vi "Boiler Controller.vi"(8 "error in":errorcluster, 10 "Notifiers":T1, 11 "Message Queues":T2) -> (0 "error out":errorcluster)   [LabVIEW 2026]
uses:
  support/Message Queue/All Message Queues.ctl
  support/Message Queue/Message Cluster.ctl
  support/Notifiers/Notifiers.ctl
  support/Message Queue/Message Queue.lvlib
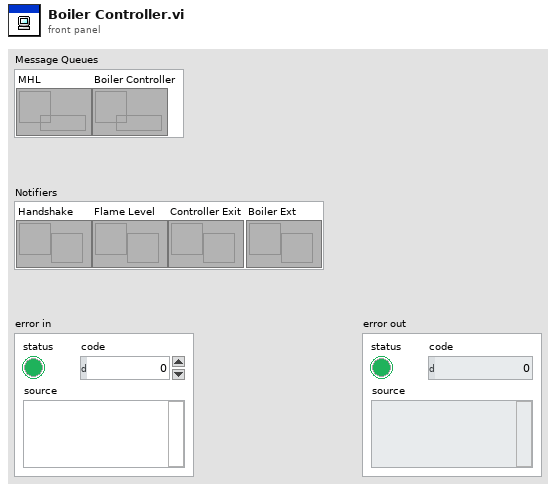
[diagram p1: front panel]
types:
  T1 = typedef "Notifiers.ctl" = cluster{"Handshake":refnum<notifier>, "Flame Level":refnum<notifier>, "Controller Exit":refnum<notifier>, "Boiler Ext":refnum<notifier>}
  T2 = typedef "Message Queue.lvlib/All Message Queues.ctl" = cluster{"MHL":refnum<queue>, "Boiler Controller":refnum<queue>}
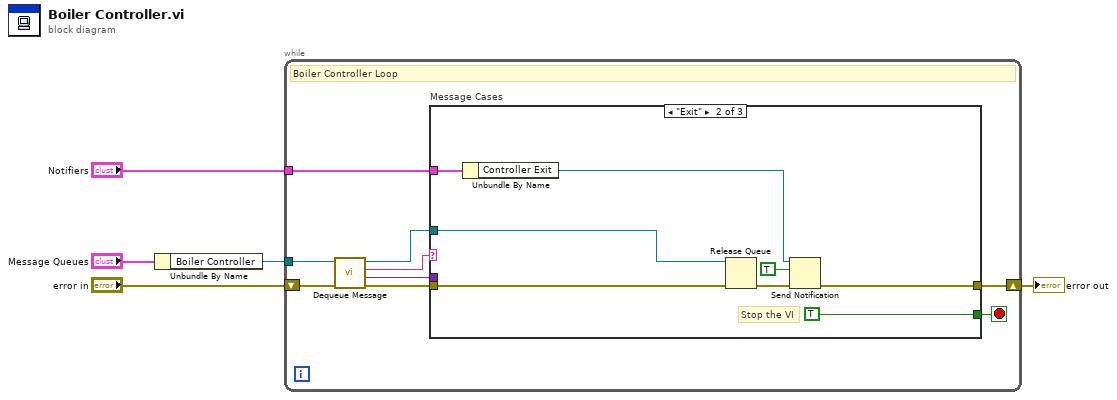
[diagram p0: block diagram]
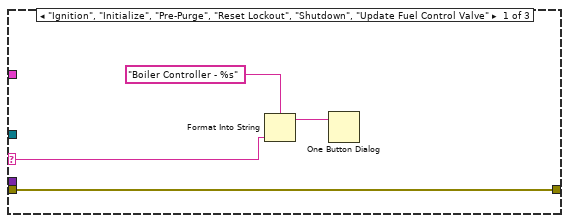
[diagram p2: hidden frame]
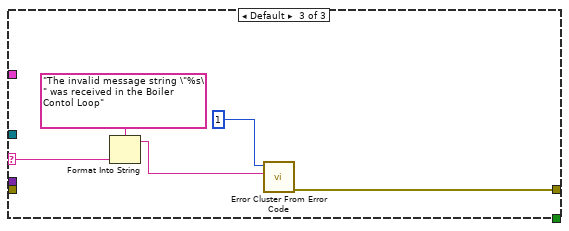
[diagram p3: hidden frame]
diagram:
  n1 = Unbundle By Name("Message Queues") -> ("Boiler Controller"=w3:refnum<queue>)
  n2 = while {
    tunnel: w3 -> [w11]
    shift-right: [w12] -> w4
    shift-left: "error in" -> [w13]
    tunnel: "Notifiers" -> [w6]
    stop <- w7 stop-if-true
    # "Boiler Controller Loop"
    n3 = call "Dequeue Message.vi"("error in"=w13, "Message Queue"=w11) -> ("error out"=w14:errorcluster, "Message Data"=w8:variant, "Message"=w10:string, "dup Message Queue"=w9:refnum<queue>)  [unwired: 6 in]
    n4 = case "Message Cases" shown="\"Exit\"" w10 {
      selector: w10 -> [w16 _ w30]
      tunnel: w9 -> [_ w23 _]
      tunnel: w8 -> [_ _ _]
      tunnel: w14 -> [w18 w26 _]
      tunnel: [w18 w24 w31] -> w12
      tunnel: [_ TRUE _] -> w7
      tunnel: w6 -> [_ w21 _]
      frame "Ignition", "Initialize", "Pre-Purge", "Reset Lockout", "Shutdown", "Update Fuel Control Valve" {
        n5 = Format Into String(format string="Boiler Controller - %s" ("message"), w16) -> (resulting string=w15:string)  [unwired: 2 in, 1 out]
        n6 = One Button Dialog(message=w15) -> ()  [unwired: 1 in, 1 out]
      }
      frame "Exit" {
        # "Stop the VI"
        n7 = Unbundle By Name(w21) -> ("Controller Exit"=w20:refnum<notifier>)
        n8 = Release Queue(queue=w23, error in (no error)=w26) -> (error out=w25:errorcluster)  [unwired: 1 in, 2 out]
        n9 = Send Notification(notification=TRUE, notifier=w20, error in (no error)=w25) -> (error out=w24:errorcluster)  [unwired: 1 out]
      }
      frame Default {
        n10 = Format Into String(format string="The invalid message string \"%s\" was received in the Boiler Contol Loop", w30) -> (resulting string=w28:string)  [unwired: 2 in, 1 out]
        n11 = call <vilib>:"Error Cluster From Error Code.vi"("error message (\"\")"=w28, "error code (0)"=1) -> ("error out"=w31:errorcluster)  [unwired: 7 in]
      }
    }
  }
  "error out" <- w4
